vi "Insight_WaveRef.vi"(6 "Gas Type":T3, 7 "Peak Fitting Controls":T2={"Pk Threshold (1 to -1)"=0.5, "Pk Fit Tol (GHz)"=2.0, "Pts to Fit at Pk"=3} {"Pts to Fit at Pk" min=3}, 8 "error in (no error)":errorcluster, 9 "Optical Freq. Step (GHz)":dbl, 10 "Start Wavelength (nm)":dbl, 11 "Gas Cell Data":dbl[](array[numeric])) -> (0 "error out":errorcluster, 1 "Best-fit Gas Cell WLs (nm)":dbl[](array[numeric]) format="%.4g", 2 "Gas Cell Locations (index)":dbl[](array[numeric]), 3 "Best Fit Wavelength Axis (nm)":dbl[](array[numeric]) format="%#.4g", 4 "First Pk Wavelength Axis (nm)":dbl[](array[numeric]) format="%#.4g", 5 "WaveRef Results":T1 {"Min Residual (pm)" format="%#.1g"; "Max Residual (pm)" format="%#.1g"; "Std Dev of Residuals (pm)" format="%0.2f"; "Mean Residual (pm)" format="%0.2f"})   [LabVIEW 2011]
doc: "Insight Photonic Solutions\n\nThis VI finds valleys in gas cell data, assigns wavelengths to the valleys, and then computes a best-fit wavelength axis to the gas cell data.\n\nINPUTS\n\nGas Type - the gas cell used (Acetylene, Hydrogen Cyanide, or Hydrogen Flouride)\nGas Cell Data - gas cell absorption data. May be in any linear units. The data are normalized from +1 to -1 inside the VI.\nStart Wavelength (nm) - estimated start wavelength of the data, based on the laser's programmed start value.\nOptical Frequency Step (GHz) - optical frequency step estimated from the laser's sweep calibration\nThreshold (+1 to -1) - Valley fit threshold, assuming that the Gas Cell Data is scaled from a max of 1 to a min of -1. In early tests, 0.5 worked well.\n\nerror in - LabView error cluster\n\nOUTPUTS\n\nBest Fit Wavelength Axis (nm) - the wavelength axis for the Gas Cell Data based on a linear fit to the Gas Cell Feature WLs\nGas Cell Locations (index) - where the VI thinks the gas cell features are in sample index\nGas Cell Feature WLs (nm) - the assigned WLs for the Gas Cell Locations\nFirst Pk Wavelength Axis (nm) - a simpler estimate of the wavelength estimate using only the first feature to pin the absolute value and the input Optical Frequency Step as the scale.\nerror out - LabView error cluster\n\nver 1.0 - original release\nver 1.1 - added Hydrogen Cyanide and Hydrogen Flouride gas cell reference lines"
uses:
  WaveRef_Gas_Types.ctl
  WaveRef Fitting Controls.ctl
  <vilib>/Analysis/baseanly.llb/Scale 1D.vi
  <vilib>/Analysis/NI_AAL_SigProc.lvlib
  <vilib>/Analysis/NI_AALBase.lvlib
  <vilib>/Analysis/NI_AALPro.lvlib
panel:
  out "Ref Lines Found":i32
  out "Total Lines Found":i32
  out "Min Residual (pm)":dbl format="%#.1g"
  out "Max Residual (pm)":dbl format="%#.1g"
  out "Std Dev of Residuals (pm)":dbl format="%0.2f"
  out "Mean Residual (pm)":dbl format="%0.2f"
  out "Gas Cell Residuals":dbl[](graph)
  out "Normalized Gas Cell Data":dbl[](graph)
  out "intercept (GHz)":dbl
  out "slope (GHz/sample)":dbl
  out "Gas Cell Feature WLs (nm)":dbl[](array[numeric]) format="%#.4g"
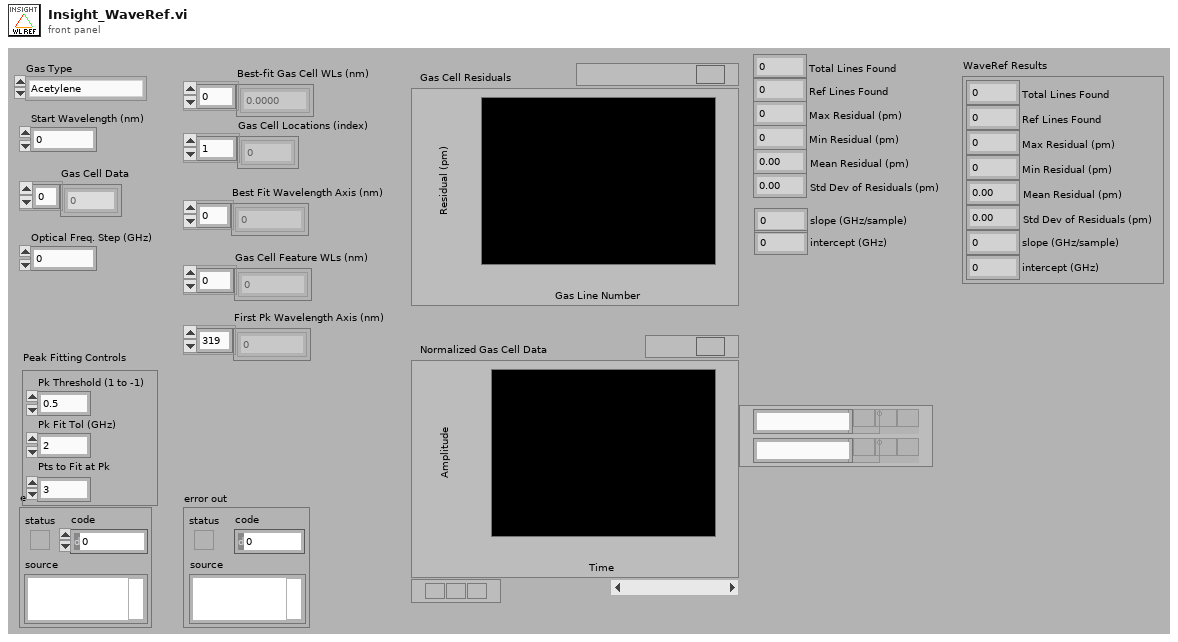
[diagram p1: front panel]
types:
  T1 = cluster{"Total Lines Found":i32, "Ref Lines Found":i32, "Max Residual (pm)":dbl, "Min Residual (pm)":dbl, "Mean Residual (pm)":dbl, "Std Dev of Residuals (pm)":dbl, "slope (GHz/sample)":dbl, "intercept (GHz)":dbl}
  T2 = typedef "WaveRef Fitting Controls.ctl" = cluster{"Pk Threshold (1 to -1)":dbl, "Pk Fit Tol (GHz)":dbl, "Pts to Fit at Pk":i32}
  T3 = typedef "WaveRef_Gas_Types.ctl" = enum16{"Acetylene", "HCN (WA-1528-1562)", "HCN (Triple Cell, WA-1520-1640)", "HCN (NIST SRM2519a)", "Hydrogen Flouride"}
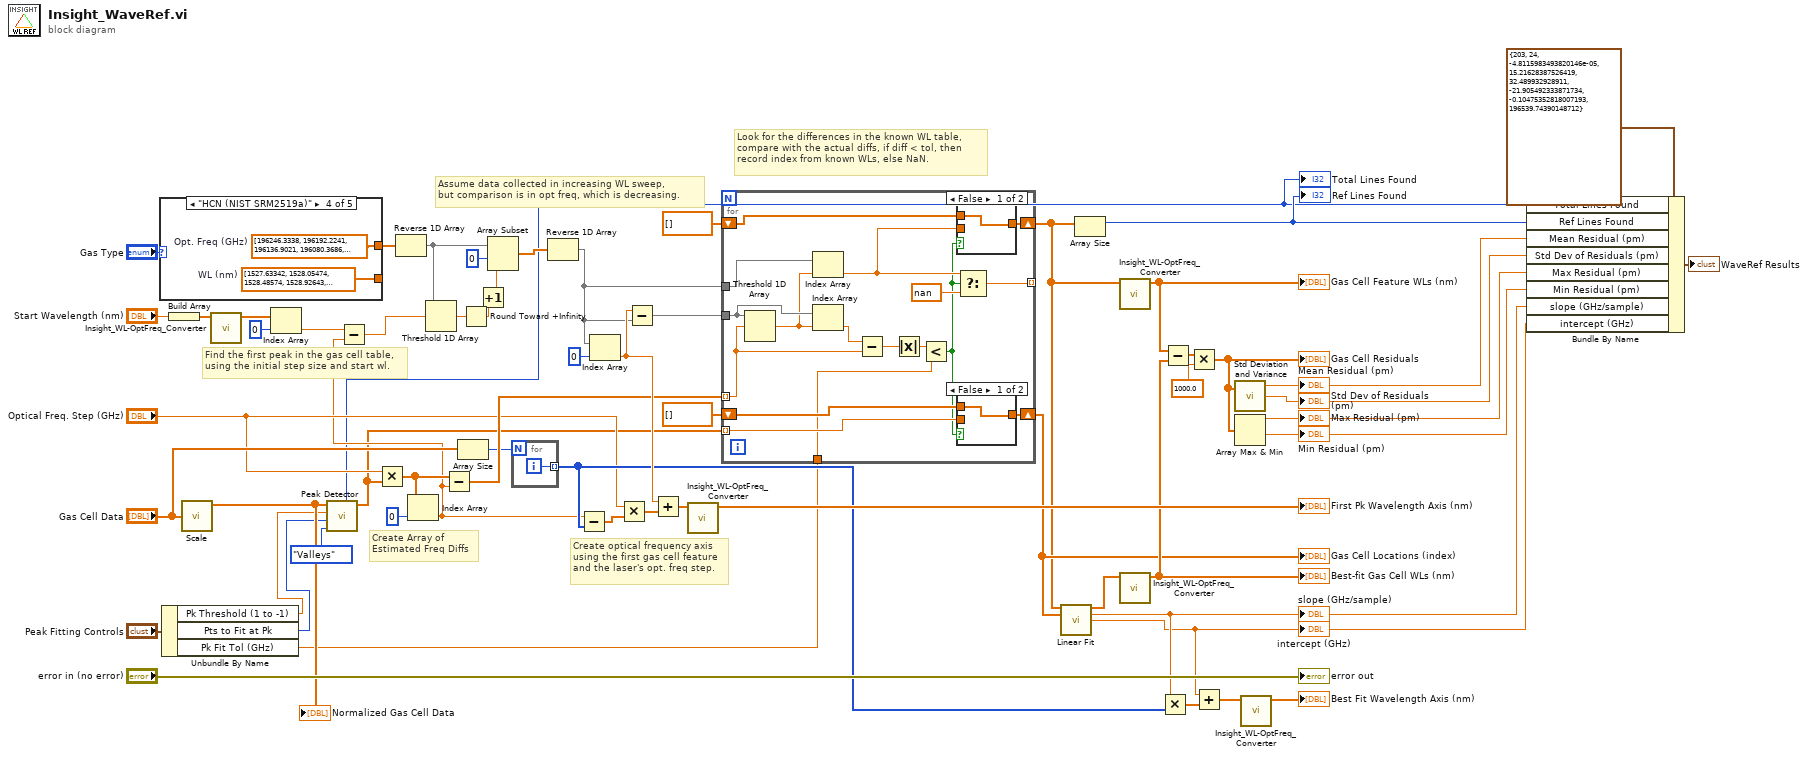
[diagram p0: block diagram]
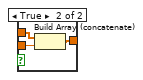
[diagram p2: hidden frame]
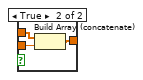
[diagram p3: hidden frame]
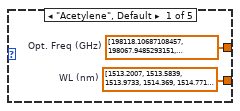
[diagram p4: hidden frame]
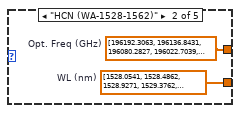
[diagram p5: hidden frame]
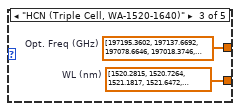
[diagram p6: hidden frame]
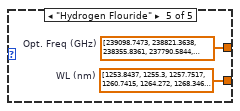
[diagram p7: hidden frame]
diagram:
  # "Find the first peak in the gas cell table,\nusing the initial step size and start wl."
  # "Look for the differences in the known WL table,\ncompare with the actual diffs, if diff < tol, then\nrecord index from known WLs, else NaN."
  # "Create optical frequency axis \nusing the first gas cell feature\nand the laser's opt. freq step."
  # "Assume data collected in increasing WL sweep,\nbut comparison is in opt freq, which is decreasing."
  # "Create Array of\nEstimated Freq Diffs"
  n1 = case shown="\"HCN (NIST SRM2519a)\"" "Gas Type" {
    tunnel: [w63 w65 w66 w68 w70] -> _
    tunnel: [w62 w64 w67 w69 w71] -> w28
    frame "Acetylene", Default {
      w62 = dbl[] [198118.10687108457, 198067.9485293151, 198017.0046591971, 197965.26341994587, 197912.72608202824, 197859.39393443402, 197805.26828459787, 197750.35045832008, 197694.65483642992, 197638.1567002801, 197580.87047437474, 197522.7975571653, 197463.92635872497, 197404.28433385078, 197343.84692999502, 197282.62862354727, 197220.63090217157, 197157.85527105053, 197094.29029511043, 197029.93753967562, 196964.8115285787, 196898.9138367592, 196832.23313296385, 196764.7710527193, 196696.5421544482, 196487.2066766433, 196415.88854513425, 196343.7991751912, 196270.94032185446, 196197.31375691248, 196122.93409907375, 196047.77748292126, 195971.85856986625, 195895.1791976303, 195817.74122014895, 195739.5465074629, 195660.58417575122, 195580.8689175951, 195500.4026509687, 195419.1745711409, 195337.1993870245, 195254.47906351043, 195171.00287477585, 195086.77284912072, 195001.80371449405, 194916.09749691008, 194829.6309139884, 194742.43138989183, 194654.48835650535, 194565.80393361207]  # Opt. Freq (GHz)
      w63 = dbl[] [1513.2007, 1513.5839, 1513.9733, 1514.369, 1514.771, 1515.1793, 1515.5939, 1516.0148, 1516.4419, 1516.8754, 1517.3152, 1517.7613, 1518.2138, 1518.6725, 1519.1376, 1519.609, 1520.0867, 1520.5707, 1521.0611, 1521.5579, 1522.061, 1522.5704, 1523.0862, 1523.6084, 1524.1369, 1525.7607, 1526.3147, 1526.8751, 1527.4419, 1528.0151, 1528.5946, 1529.1806, 1529.773, 1530.3718, 1530.977, 1531.5886, 1532.2067, 1532.8312, 1533.4621, 1534.0995, 1534.7433, 1535.3935, 1536.0502, 1536.7134, 1537.383, 1538.059, 1538.7416, 1539.4306, 1540.1261, 1540.8281]  # WL (nm)
    }
    frame "HCN (WA-1528-1562)" {
      w65 = dbl[] [1528.0541, 1528.4862, 1528.9271, 1529.3762, 1529.8376, 1530.3061, 1530.7856, 1531.2764, 1531.7738, 1532.2825, 1532.8024, 1533.3291, 1533.8671, 1534.4159, 1534.9723, 1535.5401, 1536.117, 1536.7034, 1537.2997, 1537.9069, 1538.5224, 1539.1494, 1539.7855, 1540.4314, 1541.0872, 1541.7529, 1543.1148, 1543.8094, 1544.5147, 1545.2314, 1545.9563, 1546.6902, 1547.4354, 1548.1904, 1548.9554, 1549.7302, 1550.5149, 1551.3106, 1552.1157, 1552.9308, 1553.756, 1554.5892, 1555.4346, 1556.2919, 1557.1573, 1558.0329, 1558.9185, 1559.8143, 1560.7185, 1561.6344, 1562.5625]  # WL (nm)
      w64 = dbl[] [196192.3063, 196136.8431, 196080.2827, 196022.7039, 195963.5833, 195903.5895, 195842.2251, 195779.4543, 195715.8805, 195650.9051, 195584.5437, 195517.3602, 195448.783, 195378.8787, 195308.0574, 195235.8379, 195162.5156, 195088.0424, 195012.3701, 194935.3748, 194857.3891, 194778.0105, 194697.5459, 194615.9095, 194533.092, 194449.0962, 194277.4821, 194190.0717, 194101.3951, 194011.3681, 193920.3961, 193828.3814, 193735.0393, 193640.5613, 193544.9258, 193448.1615, 193350.2593, 193251.0859, 193150.8444, 193049.4636, 192946.935, 192843.5229, 192738.7098, 192632.5376, 192525.4809, 192417.2834, 192307.9738, 192197.5315, 192086.1821, 191973.5234, 191859.4987]  # Opt. Freq (GHz)
    }
    frame "HCN (Triple Cell, WA-1520-1640)" {
      w66 = dbl[] [1520.2815, 1520.7264, 1521.1817, 1521.6472, 1522.1235, 1522.6098, 1523.1066, 1523.6138, 1524.1313, 1524.6592, 1525.1977, 1525.7467, 1526.3059, 1526.8754, 1527.4557, 1528.0462, 1528.6474, 1529.2587, 1529.8807, 1530.5133, 1531.1561, 1531.8098, 1532.474, 1535.9546, 1536.6813, 1537.42, 1538.1687, 1538.9281, 1539.6984, 1540.4791, 1541.2707, 1542.072, 1542.886, 1543.7095, 1544.5438, 1545.3888, 1546.2448, 1547.1114, 1547.9893, 1548.8773, 1549.7758, 1550.6863, 1552.5385]  # WL (nm)
      w67 = dbl[] [197195.3602, 197137.6692, 197078.6646, 197018.3746, 196956.7239, 196893.8188, 196829.5968, 196764.0737, 196697.2649, 196629.1601, 196559.7365, 196489.0096, 196417.021, 196343.7606, 196269.1671, 196193.3206, 196116.1599, 196037.7652, 195958.0626, 195877.0682, 195794.8363, 195711.2809, 195626.4563, 195183.1506, 195090.8481, 194997.1107, 194902.1964, 194806.0199, 194708.5598, 194609.8834, 194509.9313, 194408.859, 194306.2922, 194202.6385, 194097.7381, 193991.6078, 193884.2142, 193775.6118, 193665.7172, 193554.6851, 193442.4695, 193328.888, 193098.2439]  # Opt. Freq (GHz)
    }
    frame "HCN (NIST SRM2519a)" {
      w69 = dbl[] [196246.3338, 196192.2241, 196136.9021, 196080.3686, 196022.6257, 195963.6756, 195903.5178, 195842.1547, 195779.586, 195715.8166, 195650.8438, 195584.6726, 195517.3041, 195448.7384, 195378.9755, 195308.0217, 195235.8747, 195162.5372, 195088.0119, 195012.2952, 194935.3938, 194857.3068, 194778.0345, 194697.58, 194615.9348, 194533.1134, 194449.1088, 194277.5539, 194190.0377, 194101.3536, 194011.5025, 193920.4977, 193828.3375, 193735.0167, 193640.54, 193544.9071, 193448.1228, 193350.1895, 193251.1046, 193150.8742, 193049.4997, 192946.9822, 192843.3257, 192738.5301, 192632.5983, 192525.5353, 192417.3451, 192308.0256, 192197.582, 192086.0184, 191973.3353, 191859.538, 191744.6296, 191628.6105]  # Opt. Freq (GHz)
      w68 = dbl[] [1527.63342, 1528.05474, 1528.48574, 1528.92643, 1529.37681, 1529.83688, 1530.30666, 1530.78615, 1531.27537, 1531.7743, 1532.28298, 1532.80139, 1533.32954, 1533.86745, 1534.41514, 1534.97258, 1535.53981, 1536.11683, 1536.70364, 1537.30029, 1537.90675, 1538.52305, 1539.14921, 1539.78523, 1540.4312, 1541.08703, 1541.7528, 1543.11423, 1543.80967, 1544.51503, 1545.23033, 1545.95549, 1546.69055, 1547.43558, 1548.19057, 1548.95555, 1549.73051, 1550.51546, 1551.31045, 1552.11546, 1552.93051, 1553.75562, 1554.59079, 1555.43605, 1556.29141, 1557.15686, 1558.0324, 1558.91808, 1559.81389, 1560.71983, 1561.63593, 1562.56218, 1563.49859, 1564.44519]  # WL (nm)
    }
    frame "Hydrogen Flouride" {
      w70 = dbl[] [1253.8437, 1255.3, 1257.7517, 1260.7415, 1264.272, 1268.3468, 1272.9703, 1278.1478, 1283.8856, 1297.07, 1304.5337, 1312.5909, 1321.2524, 1330.5299, 1340.4363, 1350.9856, 1362.193]  # WL (nm)
      w71 = dbl[] [239098.7473, 238821.3638, 238355.8361, 237790.5844, 237126.5503, 236364.7372, 235506.2471, 234552.2623, 233504.0272, 231130.5157, 229808.136, 228397.4832, 226900.2183, 225318.0917, 223652.8942, 221906.4792, 220080.7507]  # Opt. Freq (GHz)
    }
  }
  n2 = Unbundle By Name("Peak Fitting Controls") -> ("Pk Threshold (1 to -1)"=w12:dbl, "Pts to Fit at Pk"=w13:i32, "Pk Fit Tol (GHz)"=w11:dbl)
  n3 = Build Array("Start Wavelength (nm)") -> (w35:dbl[])
  n4 = call-poly <vilib>:"Scale.vi"("X"="Gas Cell Data") -> ("Y=(X-offset)/scale"=w43:dbl[])  [unwired: 3 out]
  "Normalized Gas Cell Data" <- w43
  n5 = call "Insight_WL-OptFreq_Converter.vi"("WL or Opt. Freq"=w35) -> ("Opt. Freq or WL"=w33:dbl[])  [unwired: 9 in, 1 out]
  n6 = Index Array(array=w33, index=0) -> (element=w27:dbl)
  n7 = call <vilib>:"Peak Detector.vi"("peaks/valleys"=enum32{"Peaks", "Valleys"}."Valleys", "width"=w13, "threshold"=w12, "X"=w43) -> ("Locations"=w20:dbl[], "# found"=w9:i32)  [unwired: 3 in, 3 out]
  "Total Lines Found" <- w9
  n8 = Multiply(x="Optical Freq. Step (GHz)", y=w20) -> (x*y=w42:dbl[])
  n9 = Reverse 1D Array(array=w28) -> (reversed array=w26:dbl[])
  n10 = Index Array(array=w42, index=0) -> (element=w31:dbl)
  n11 = Subtract(x=w27, y=w31) -> (x-y=w22:dbl)
  n12 = Threshold 1D Array(2:w22, 3:w26) -> (0:w58:dbl)  [unwired: 1 in]
  n13 = Subtract(x=w42, y=w31) -> (x-y=w54:dbl[])
  n14 = Array Size(array="Gas Cell Data") -> (size(s)=w47:i32)
  n15 = Round Toward +Infinity(x=w58) -> (ceil(x): smallest int >= x=w23:dbl)
  n16 = Increment(x=w23) -> (x+1=w21:dbl)
  n17 = Array Subset(array=w26, index=0, length=w21) -> (w29:dbl[])
  n18 = for {
    N: w47 -> [_]
    tunnel: [w72] -> w46 mode=indexing
    i -> [w72]
  }
  n19 = Reverse 1D Array(array=w29) -> (reversed array=w25:dbl[])
  n20 = Subtract(x=w31, y=w46) -> (x-y=w49:dbl[])
  n21 = Index Array(array=w25, index=0) -> (element=w55:dbl)
  n22 = Multiply(x="Optical Freq. Step (GHz)", y=w49) -> (x*y=w48:dbl[])
  n23 = Subtract(x=w55, y=w25) -> (x-y=w41:dbl[])
  n24 = Add(x=w55, y=w48) -> (x+y=w53:dbl[])
  n25 = call "Insight_WL-OptFreq_Converter.vi"("WL or Opt. Freq"=w53) -> ("Opt. Freq or WL"=→"First Pk Wavelength Axis (nm)":dbl[])  [unwired: 9 in, 1 out]
  n26 = for {
    tunnel: w54 -> [w88] mode=indexing
    tunnel: w41 -> [w89]
    tunnel: w25 -> [w85]
    tunnel: [w83] -> _ mode=indexing
    tunnel: w20 -> [w80] mode=indexing
    shift-right: [w79] -> w17
    shift-left: dbl[] [] -> [w78]
    shift-right: [w77] -> w16
    shift-left: dbl[] [] -> [w74]
    tunnel: w11 -> [w73]
    n27 = Threshold 1D Array(2:w88, 3:w89) -> (0:w81:dbl)  [unwired: 1 in]
    n28 = Index Array(array=w85, index=w81) -> (element=w76:dbl)
    n29 = Index Array(array=w89, index=w81) -> (element=w86:dbl)
    n30 = Subtract(x=w86, y=w88) -> (x-y=w82:dbl)
    n31 = Absolute Value(x=w82) -> (abs(x)=w87:dbl)
    n32 = Less?(x=w87, y=w73) -> (x < y?=w75:bool)
    n33 = case shown="False" w75 {
      tunnel: w76 -> [_ w93]
      tunnel: [w90 w92] -> w77
      tunnel: w74 -> [w90 w91]
      frame False {
      }
      frame True {
        n34 = Build Array (concatenate)(w91, w93) -> (w92:dbl[])
      }
    }
    n35 = case shown="False" w75 {
      tunnel: w80 -> [_ w97]
      tunnel: [w94 w96] -> w79
      tunnel: w78 -> [w94 w95]
      frame False {
      }
      frame True {
        n36 = Build Array (concatenate)(w95, w97) -> (w96:dbl[])
      }
    }
    n37 = Select(t=w76, s=w75, f=nan) -> (s? t:f=w83:dbl)
  }
  "Gas Cell Locations (index)" <- w17
  n38 = call <vilib>:"Linear Fit.vi"("Y"=w16, "X"=w17) -> ("Best Linear Fit"=w51:dbl[], "slope"=w4:dbl, "intercept"=w3:dbl)  [unwired: 9 in, 2 out]
  "slope (GHz/sample)" <- w4
  "intercept (GHz)" <- w3
  n39 = Array Size(array=w16) -> (size(s)=w10:i32)
  "Ref Lines Found" <- w10
  n40 = call "Insight_WL-OptFreq_Converter.vi"("WL or Opt. Freq"=w16) -> ("Opt. Freq or WL"=w40:dbl[])  [unwired: 9 in, 1 out]
  "Gas Cell Feature WLs (nm)" <- w40
  n41 = call "Insight_WL-OptFreq_Converter.vi"("WL or Opt. Freq"=w51) -> ("Opt. Freq or WL"=w39:dbl[])  [unwired: 9 in, 1 out]
  "Best-fit Gas Cell WLs (nm)" <- w39
  n42 = Multiply(x=w4, y=w46) -> (x*y=w50:dbl[])
  n43 = Subtract(x=w40, y=w39) -> (x-y=w38:dbl[])
  n44 = Multiply(x=w38, y=1000.0) -> (x*y=w36:dbl[])
  "Gas Cell Residuals" <- w36
  n45 = Add(x=w3, y=w50) -> (x+y=w45:dbl[])
  n46 = call <vilib>:"Std Deviation and Variance.vi"("X"=w36) -> ("mean"=w8:dbl, "standard deviation"=w7:dbl)  [unwired: 1 in, 1 out]
  "Mean Residual (pm)" <- w8
  "Std Dev of Residuals (pm)" <- w7
  n47 = Array Max & Min(array=w36) -> (max value=w6:dbl, min value=w5:dbl)  [unwired: 2 out]
  "Max Residual (pm)" <- w6
  "Min Residual (pm)" <- w5
  n48 = call "Insight_WL-OptFreq_Converter.vi"("WL or Opt. Freq"=w45) -> ("Opt. Freq or WL"=→"Best Fit Wavelength Axis (nm)":dbl[])  [unwired: 9 in, 1 out]
  n49 = Bundle By Name(cluster=T1 {"Total Lines Found"=203, "Ref Lines Found"=24, "Max Residual (pm)"=-4.8115983493820146e-05, "Min Residual (pm)"=15.21628387526419, "Mean Residual (pm)"=32.489932928911, "Std Dev of Residuals (pm)"=-21.905492333871734, "slope (GHz/sample)"=-0.10475352818007193, "intercept (GHz)"=196539.74390148712} ("WaveRef Results"), "Total Lines Found"=w9, "Ref Lines Found"=w10, "Mean Residual (pm)"=w8, "Std Dev of Residuals (pm)"=w7, "Max Residual (pm)"=w6, "Min Residual (pm)"=w5, "slope (GHz/sample)"=w4, "intercept (GHz)"=w3) -> (→"WaveRef Results":T1)
  "error out" <- "error in (no error)"
